vi "DeInit.vi"(8 "error in":errorcluster, 11 "Plugin_Controller in":refnum<class "Plugin_Controller.lvclass">) -> (0 "error out":errorcluster, 3 "Plugin_Controller out":refnum<class "Plugin_Controller.lvclass">)   [LabVIEW 2020, in "Plugin.lvlib" / "Plugin_Controller.lvclass"]
doc: "Closes the connection."
uses:
  Plugin_Controller.lvclass
  C:/SVN_LabSys/labsys_lvcode/LabSys_SourceCode/builds/Libraries/LabSys Framework.lvlibp/Configurable Data Node/Configurable Data Node/Configurable Data Node.lvclass
  Plugin_Controller.lvclass/Plugin_Controller.ctl
  builds/Libraries/LabSys Framework.lvlibp/Configurable Data Node/Configurable Data Node/Read Module Configuration.vi
  builds/Libraries/LabSys Framework.lvlibp/Configuration Storage/Module Configuration/Module Configuration.lvclass
  Channels/Output Channels/Output Channels.lvclass
  UI_Class/Plugin_UI.lvclass
  Plugin_Driver/Plugin_Driver.lvclass
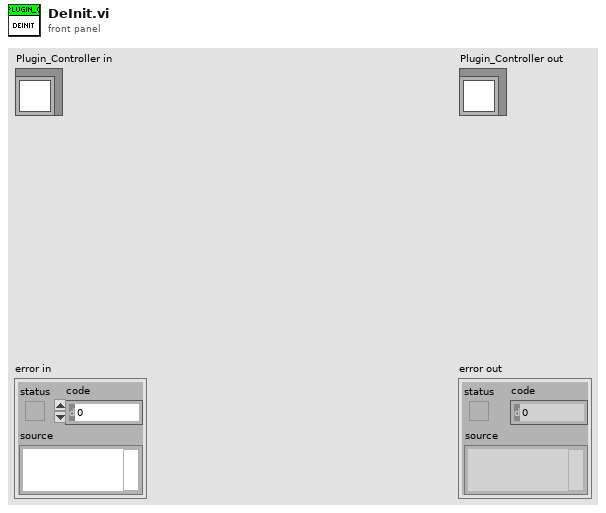
[diagram p1: front panel]
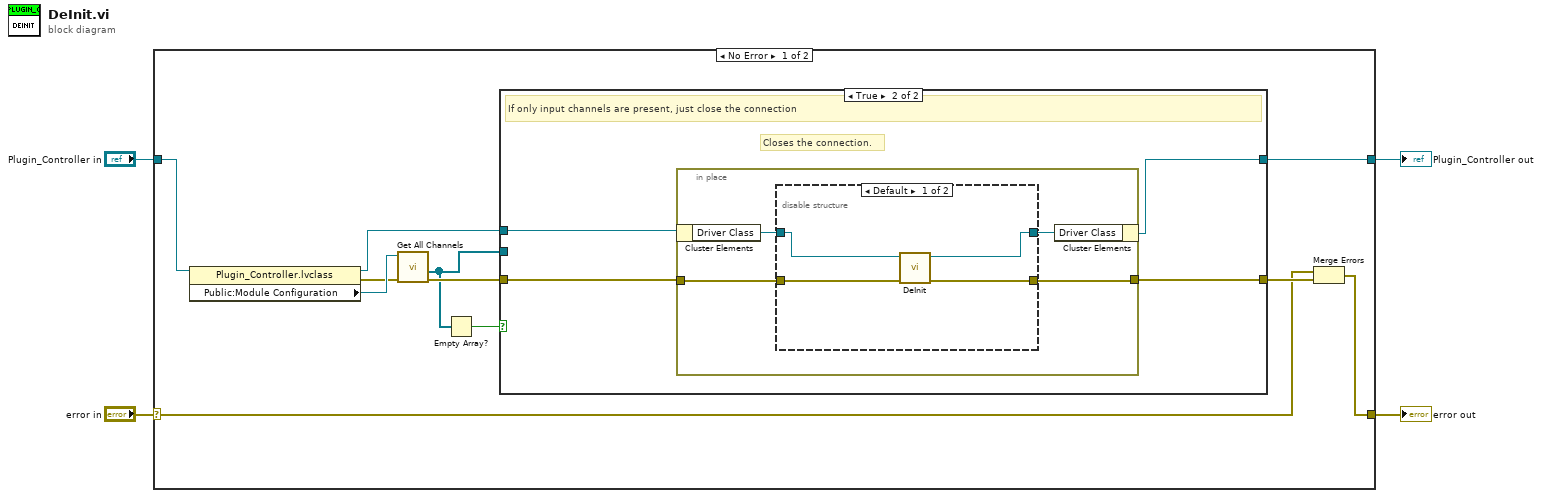
[diagram p0: block diagram]
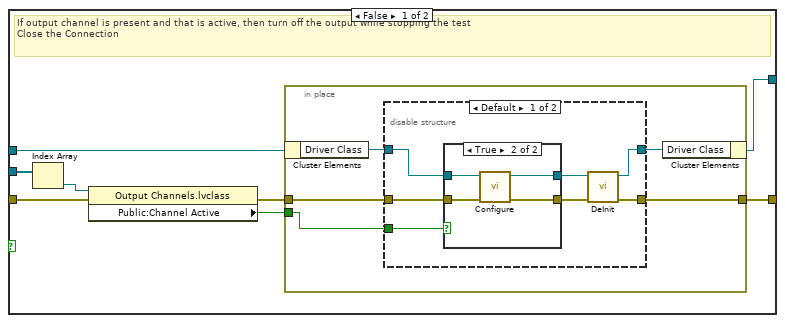
[diagram p2: hidden frame]
diagram:
  n1 = case shown="No Error" "error in" {
    selector: "error in" -> [w5 w58]
    tunnel: "Plugin_Controller in" -> [w11 w59]
    tunnel: [w10 w59] -> w3
    tunnel: [w8 w58] -> w2
    frame No Error {
      n2 = property on="Property Node" class="Plugin_Controller.lvclass"(reference=w11) -> (reference out=w12:refnum<class "Plugin_Controller.lvclass">, error out=w14:errorcluster, "Public:Module Configuration"=w15:refnum<class "Module Configuration.lvclass">)  [unwired: 1 in]
      n3 = call "Get All Channels.vi"("error in (no error)"=w14, "Module Configuration"=w15) -> ("error out"=w13:errorcluster, "Output Channels[]"=w7:refnum<class "Output Channels.lvclass">[])  [unwired: 5 in, 3 out]
      n4 = Empty Array?(array=w7) -> (empty?=w6:bool)
      n5 = case shown="True" w6 {
        tunnel: w13 -> [w16 w46]
        tunnel: w12 -> [w22 w47]
        tunnel: [w19 w45] -> w10
        tunnel: [w18 w44] -> w9
        tunnel: w7 -> [w17 _]
        frame False {
          # "If output channel is present and that is active, then turn off the output while stopping the test\nClose the Connection"
          n6 = Index Array(array=w17) -> (element=w23:refnum<class "Output Channels.lvclass">)  [unwired: 1 in]
          n7 = property on="Property Node" class="Output Channels.lvclass"(reference=w23, error in=w16) -> (error out=w21:errorcluster, "Public:Channel Active"=w20:bool)  [unwired: 1 out]
          n8 = in-place "In Place Element Structure" {
            in-place-border: w21 -> [w28]
            in-place-border: w20 -> [w26]
            in-place-border: [w24] -> w18
            n9 = in-place-cluster #1(w22) -> ("Driver Class"=w27:refnum<class "Plugin_Driver.lvclass">)
            n10 = disable-structure "Conditional Disable Structure" shown="Default" {
              disable-tunnel: w28 -> [w35 w42]
              disable-tunnel: w27 -> [w34 w43]
              disable-tunnel: w26 -> [w33 _]
              disable-tunnel: [w30 w43] -> w25
              disable-tunnel: [w29 w42] -> w24
              frame condition #0 (active) {
                n11 = case shown="True" w33 {
                  tunnel: w35 -> [w36 w41]
                  tunnel: w34 -> [w37 w40]
                  tunnel: [w36 w39] -> w31
                  tunnel: [w37 w38] -> w32
                  frame False {
                  }
                  frame True {
                    n12 = call "Configure.vi"("error in"=w41, "Plugin_Driver in"=w40) -> ("error out"=w39:errorcluster, "Plugin_Driver out"=w38:refnum<class "Plugin_Driver.lvclass">)  [unwired: 8 in]
                  }
                }
                n13 = call "DeInit.vi"("error in"=w31, "Plugin_Driver in"=w32) -> ("error out"=w29:errorcluster, "Plugin_Driver out"=w30:refnum<class "Plugin_Driver.lvclass">)  [unwired: 8 in]
              }
              frame condition #1 {
              }
            }
            n14 = in-place-cluster #1("Driver Class"=w25) -> (w19:refnum<class "Plugin_Controller.lvclass">)
          }
        }
        frame True {
          # "Closes the connection."
          # "If only input channels are present, just close the connection"
          n15 = in-place "In Place Element Structure" {
            in-place-border: w46 -> [w51]
            in-place-border: [w48] -> w44
            n16 = in-place-cluster #2(w47) -> ("Driver Class"=w50:refnum<class "Plugin_Driver.lvclass">)
            n17 = disable-structure "Conditional Disable Structure" shown="Default" {
              disable-tunnel: w51 -> [w55 w56]
              disable-tunnel: w50 -> [w54 w57]
              disable-tunnel: [w53 w57] -> w49
              disable-tunnel: [w52 w56] -> w48
              frame condition #0 (active) {
                n18 = call "DeInit.vi"("error in"=w55, "Plugin_Driver in"=w54) -> ("error out"=w52:errorcluster, "Plugin_Driver out"=w53:refnum<class "Plugin_Driver.lvclass">)  [unwired: 8 in]
              }
              frame condition #1 {
              }
            }
            n19 = in-place-cluster #2("Driver Class"=w49) -> (w45:refnum<class "Plugin_Controller.lvclass">)
          }
        }
      }
      n20 = Merge Errors(w5, w9) -> (w8:errorcluster)
    }
    frame Error {
    }
  }
  "error out" <- w2
  "Plugin_Controller out" <- w3
